vi "Get Angle.vi"(11 "arm in":refnum<class "arm.lvclass">) -> (2 "Angle":dbl, 3 "arm out":refnum<class "arm.lvclass">)   [LabVIEW 2015, in "arm.lvclass"]
uses:
  arm.lvclass
  arm.lvclass/arm.ctl
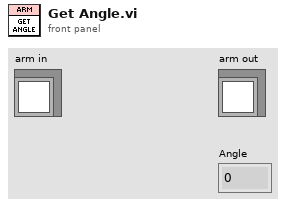
[diagram p1: front panel]
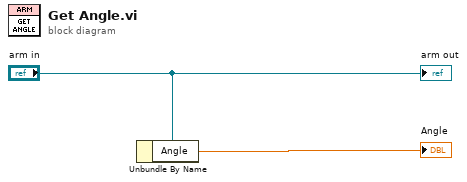
[diagram p0: block diagram]
diagram:
  n1 = Unbundle By Name("arm in") -> ("Angle"=→"Angle":dbl)
  "arm out" <- "arm in"
